vi "Stop Core.vi"(10 "final error code":i32, 11 "Network Actor in":refnum<class "Client Proxy LNA.lvclass">) -> (3 "Network Actor out":refnum<class "Client Proxy LNA.lvclass">)   [LabVIEW 2026, in "Client Proxy LNA.lvlib" / "Client Proxy LNA.lvclass"]
doc: "Defines what the actor does before it stops. Use the <B>final error code</B> input to determine whether the actor shut down normally. By default, a value of 43 indicates the actor stopped normally. Any other value indicates the actor stopped due to an error. However, descendants of Actor.lvclass can override Actor.lvclass:Handle Error.vi to change this behavior.\n\nBy default, this method does nothing. A descendant class may override it to define behavior, such as shutting down any processes the actor initiated in its override of Actor.lvclass:Actor Core.vi."
uses:
  Client Proxy LNA.lvclass
  C:/Program Files/National Instruments/LabVIEW 2026/vi.lib/ActorFramework/Actor/Actor.lvclass
  <vilib>/ActorFramework/Actor/Actor.lvclass/Actor.ctl
  Controller/Messages/Client Disconnected Msg/Client Disconnected Msg.lvclass/Client Disconnected Msg.ctl
  <vilib>/ActorFramework/Message Enqueuer/Message Enqueuer.lvclass/Message Enqueuer.ctl
  <vilib>/ActorFramework/Message Enqueuer/Enqueue.vi
  Controller/Messages/Client Disconnected Msg/Client Disconnected Msg.lvclass
  C:/Program Files/National Instruments/LabVIEW 2026/vi.lib/ActorFramework/Message/Message.lvclass
  <vilib>/ActorFramework/Message Priority Queue/Priority Enqueue.vi
  recovery/packages/ni_lib_linked_network_actor-1.2.0.19-9492AF5A82/File Group 0/vi.lib/NI/Actors/Linked Network Actor/Linked Network Actor/Linked Network Actor.lvclass
  <vilib>/ActorFramework/Actor/Actor.lvclass
  MAL-Framework/user.lib/Common Components/Controller/Messages/Log Status/Log Status.lvclass
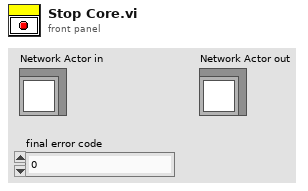
[diagram p1: front panel]
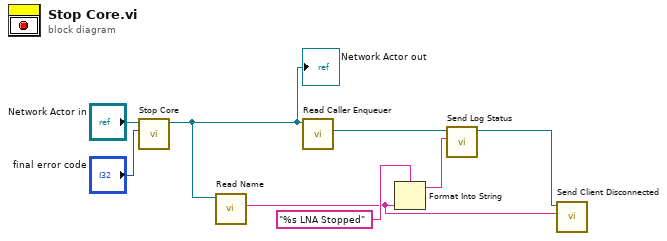
[diagram p0: block diagram]
diagram:
  n1 = call-parent "Stop Core.vi"("final error code"="final error code", "Network Actor in"="Network Actor in") -> ("Network Actor out"=w1:refnum<class "Client Proxy LNA.lvclass">)  [unwired: 9 in]
  "Network Actor out" <- w1
  n2 = call-dynamic "Read Name.vi"("Network Actor in"=w1) -> ("Name"=w3:string)  [unwired: 10 in]
  n3 = call <vilib>:"Read Caller Enqueuer.vi"("Actor"=w1) -> ("Caller Enqueuer"=w5:refnum<class "Message Enqueuer.lvclass">)  [unwired: 10 in]
  n4 = Format Into String(format string="%s LNA Stopped", w3) -> (resulting string=w4:string)  [unwired: 2 in, 1 out]
  n5 = call "Send Log Status.vi"("String"=w4, "Message Enqueuer in"=w5) -> ("Message Enqueuer out"=w2:refnum<class "Message Enqueuer.lvclass">)  [unwired: 8 in, 1 out]
  n6 = call "Send Client Disconnected.vi"("ConnectionID"=w3, "Message Enqueuer"=w2) -> ()  [unwired: 8 in, 2 out]
